vi "Read SystemConfig.vi"(8 "error in (no error)":errorcluster, 11 "SystemConfiguration in":refnum<class "SystemConfiguration.lvclass">) -> (0 "error out":errorcluster, 2 "SystemConfig":T1, 3 "SystemConfiguration out":refnum<class "SystemConfiguration.lvclass">)   [LabVIEW 2019, in "SystemSetup.lvlib" / "SystemConfiguration.lvclass"]
uses:
  SystemConfiguration.lvclass
  SystemConfig.ctl
  SystemConfiguration.lvclass/SystemConfiguration.ctl
  SystemSetup.lvclass
panel:
  # "StationInfo"
  # "SaveDataPath"
  # "TestStand"
  # "CurrentImage"
  # "BarCodeScanner"
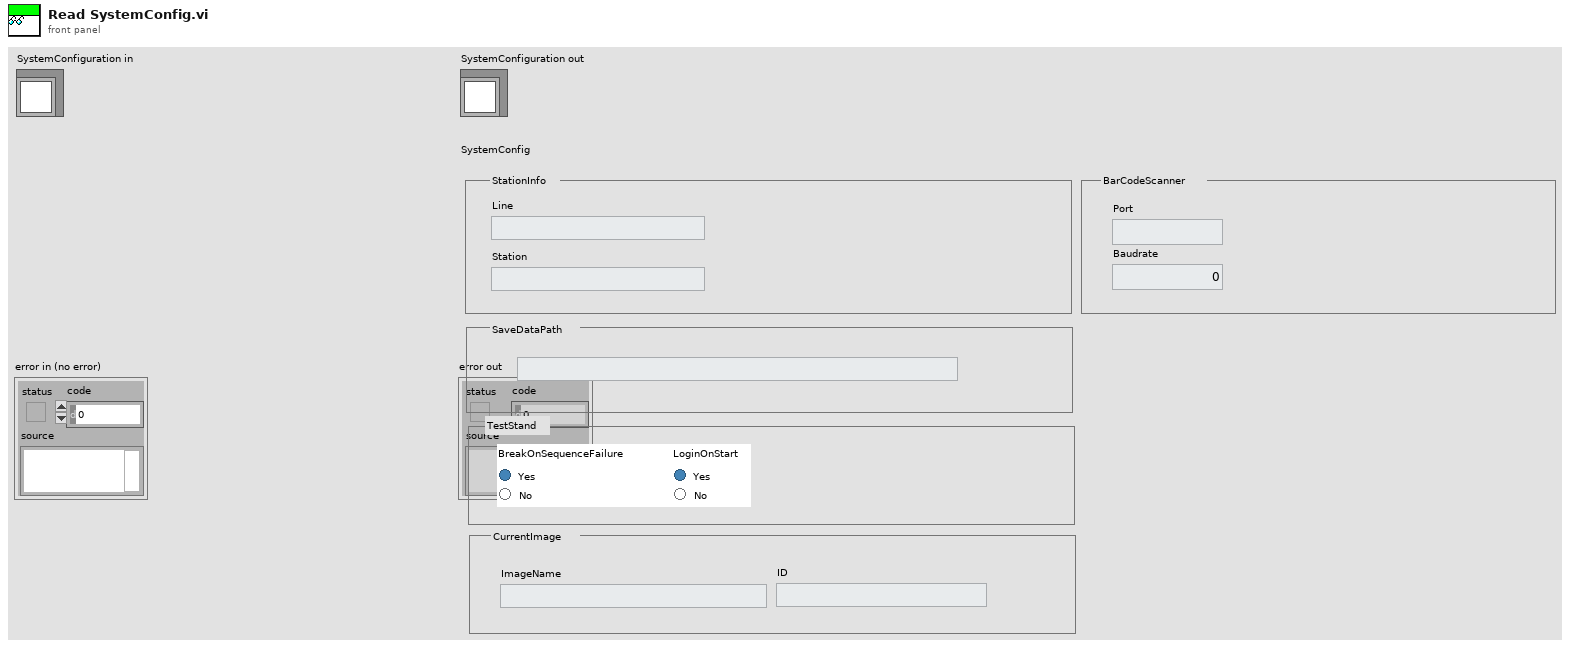
[diagram p1: front panel]
types:
  T1 = typedef "SystemSetup.lvlib/SystemSetup.lvclass/SystemConfig.ctl" = cluster{"StationInfo":cluster{"Line":string, "Station":string}, "SaveDataPath":cluster{"Path":path}, "TestStand":cluster{"BreakOnSequenceFailure":enum32{"Yes", "No"}, "LoginOnStart":enum32{"Yes", "No"}}, "CurrentImage":cluster{"ImageName":string, "ID":string}, "HardwareConfiguration":cluster{"BarCodeScanner":cluster{"Port":string, "Baudrate":i32}}}
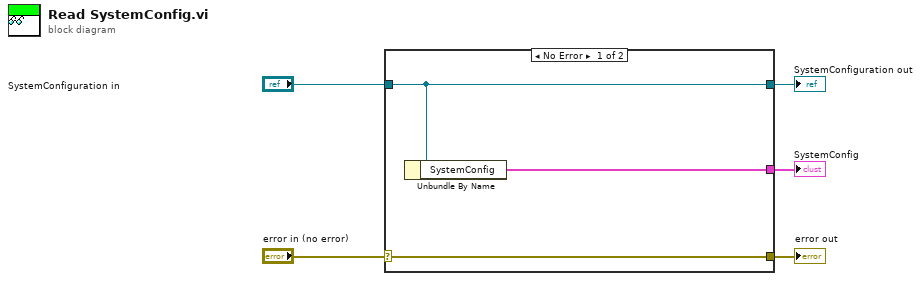
[diagram p0: block diagram]
diagram:
  n1 = case shown="No Error" "error in (no error)" {
    selector: "error in (no error)" -> [w8 w9]
    tunnel: [w8 w9] -> w4
    tunnel: [w7 w10] -> w2
    tunnel: "SystemConfiguration in" -> [w7 w10]
    tunnel: [w6 _] -> w1
    frame No Error {
      n2 = Unbundle By Name(w7) -> ("SystemConfig"=w6:T1)
    }
    frame Error {
    }
  }
  "error out" <- w4
  "SystemConfiguration out" <- w2
  "SystemConfig" <- w1
